vi "Mindsensors LineLeader Config.vi"(10 "Node Data":T1, 11 "NXT":T2) -> ()   [LabVIEW 2010]
uses:
  <vilib>/NXT/Subs/LVHSConnector.ctl
  Datatypes/Node.ctl
  UI Controls/PlugInControls/Pluginbackground.ctl
  <vilib>/Utility/miscctls.llb/LVPointTypeDef.ctl
  ConvertNodeAddrSensor.vi
panel:
  in  "Device Address":u8=2 format="%x"
  out "NXT Port":dbl format="%#.2g"
  out "S 8":dbl
  out "S 7":dbl
  out "S 6":dbl
  out "S 5":dbl
  out "S 4":dbl
  out "S 2":dbl
  out "S 3":dbl
  out "S 1":dbl
  out "XY Graph":cluster{i32[], "data Buffer":u8[]}(graph)
  out "Boolean array":bool[](array[boolean])
  in  "Name":string
  out "Headline":string="Type (auto populated)"
  in  "Sensor parameters":string
  in  "Instance Specific Data":cluster{"Example Data":dbl}
  in  "Reset":bool
  in  "Save":bool
  in  "Stop":bool
  out "Background":T3=TRUE
  # "<- No controls below this line"
  # "Common controls such as Buttons, Rings, Sliders, Graphs, Decorations, etc can be found in the <labview>\\Targets\\NI\\NXT\\NXT Toolkit\\Schematic Editor\\UI Controls\\Plugin Controls\\ folder. Use these controls when possible to ensure a consistent look and feel with LabVIEW Education Edition."
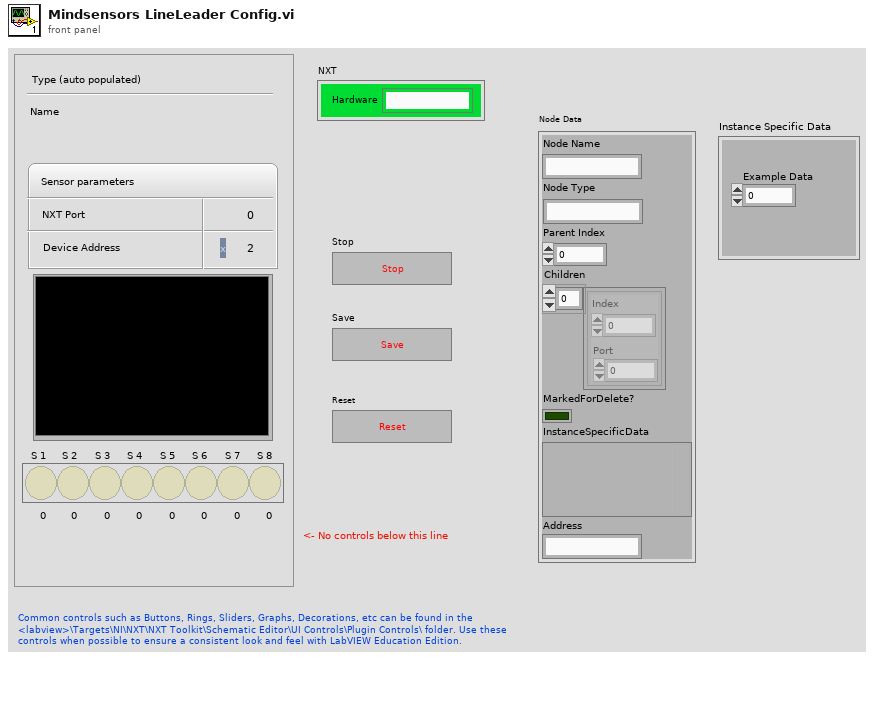
[diagram p1: front panel]
types:
  T1 = typedef "Node.ctl" = cluster{"Node Name":string, "Node Type":string, "Parent Index":i16, "Children":cluster{"Index":u16, "Port":u16}[], "MarkedForDelete?":bool, "InstanceSpecificData":variant, "Address":string}
  T2 = typedef "LVHSConnector.ctl" = cluster{"Hardware":string, "Flattened String":string}
  T3 = typedef "Pluginbackground.ctl" = bool
  T4 = typedef "LVPointTypeDef.ctl" = cluster{"Horizontal":i16, "Vertical":i16}
  T5 = enum8{"Enabled", "Disabled", "Disabled and Grayed Out"}
  T6 = typedef "NXT_InputPort.ctl" = u8
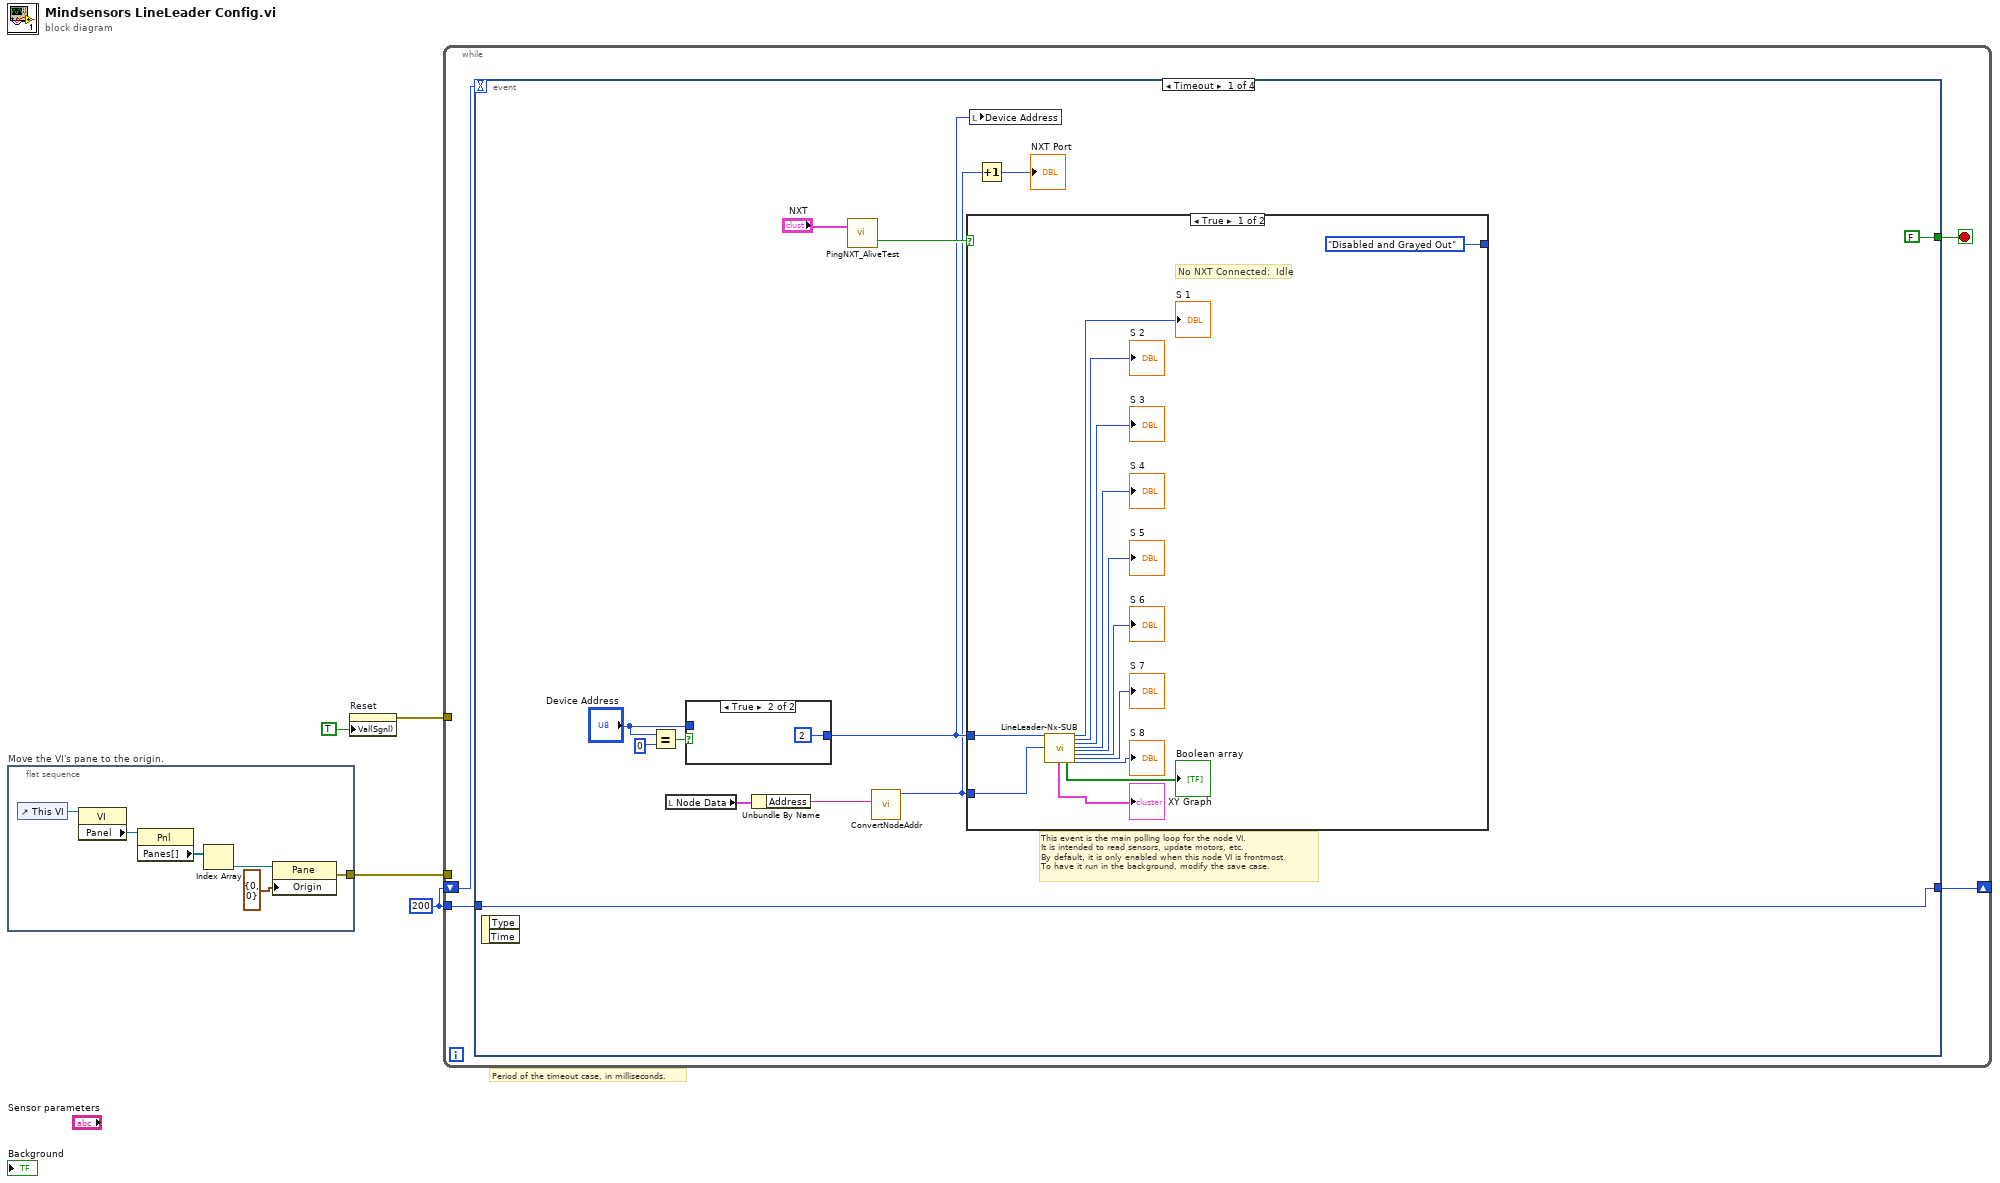
[diagram p0: block diagram]
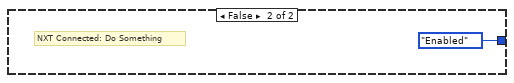
[diagram p3: hidden frame]
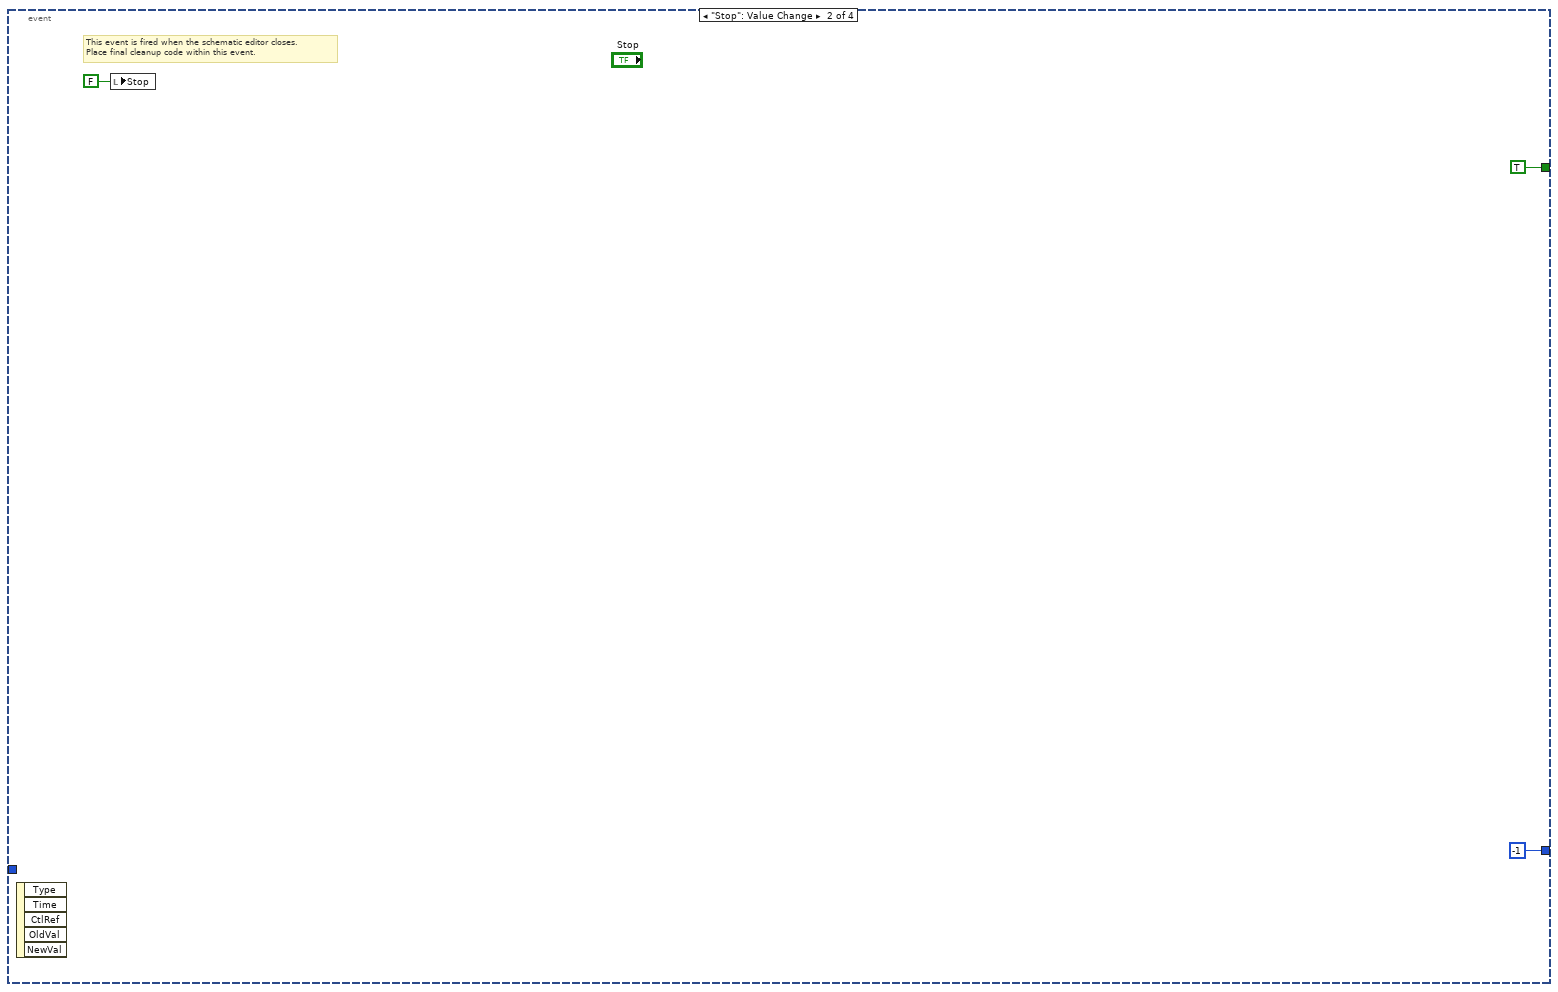
[diagram p4: hidden frame]
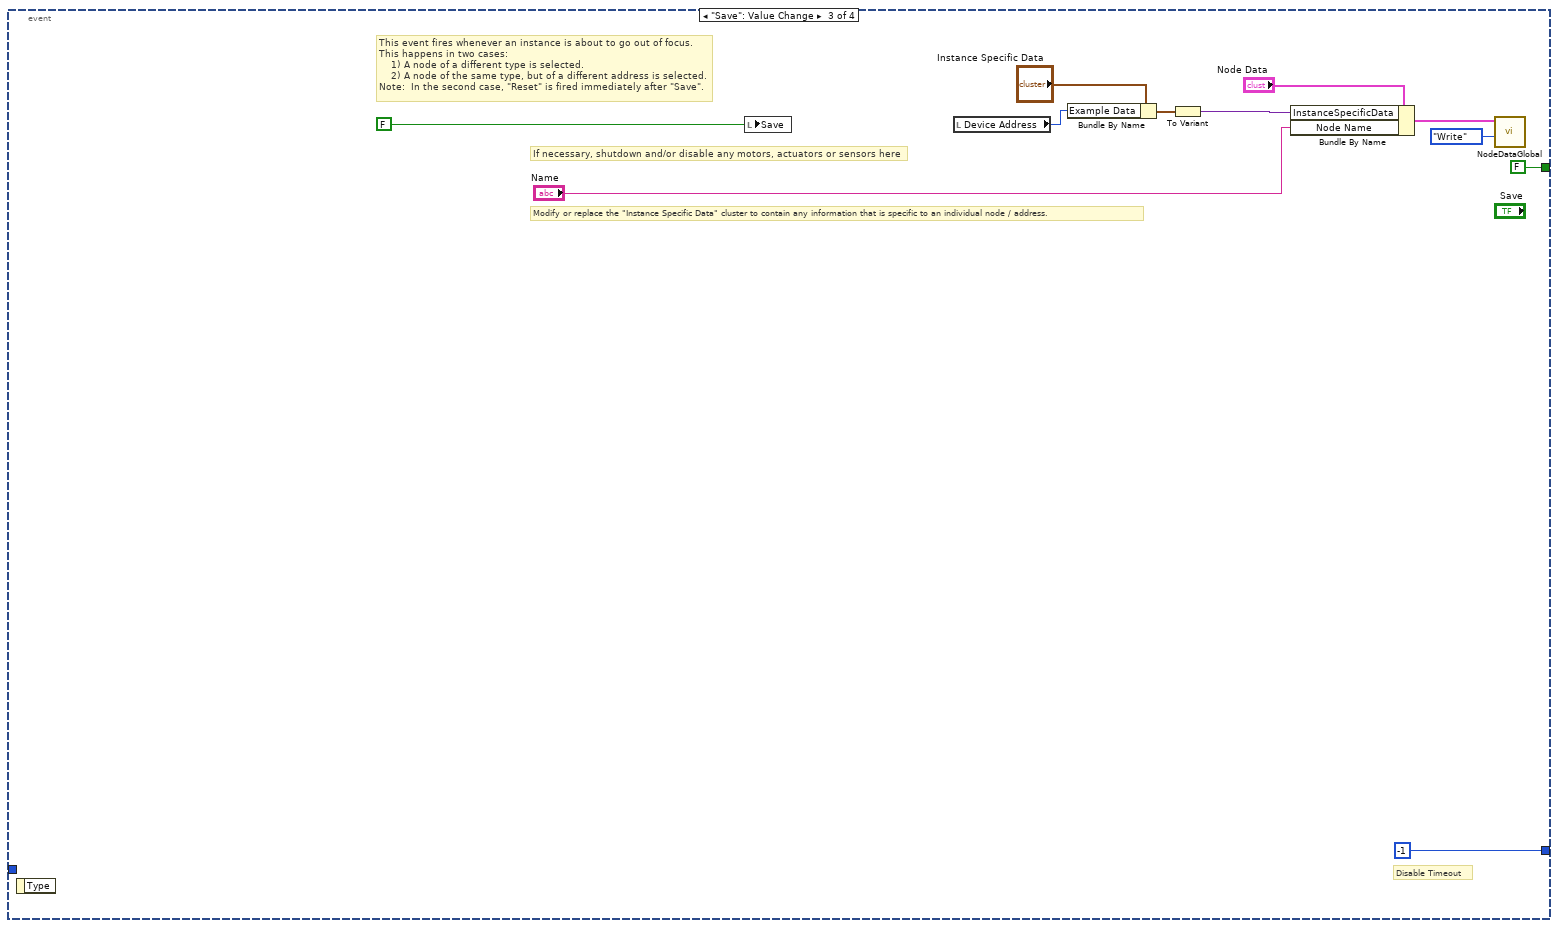
[diagram p5: hidden frame]
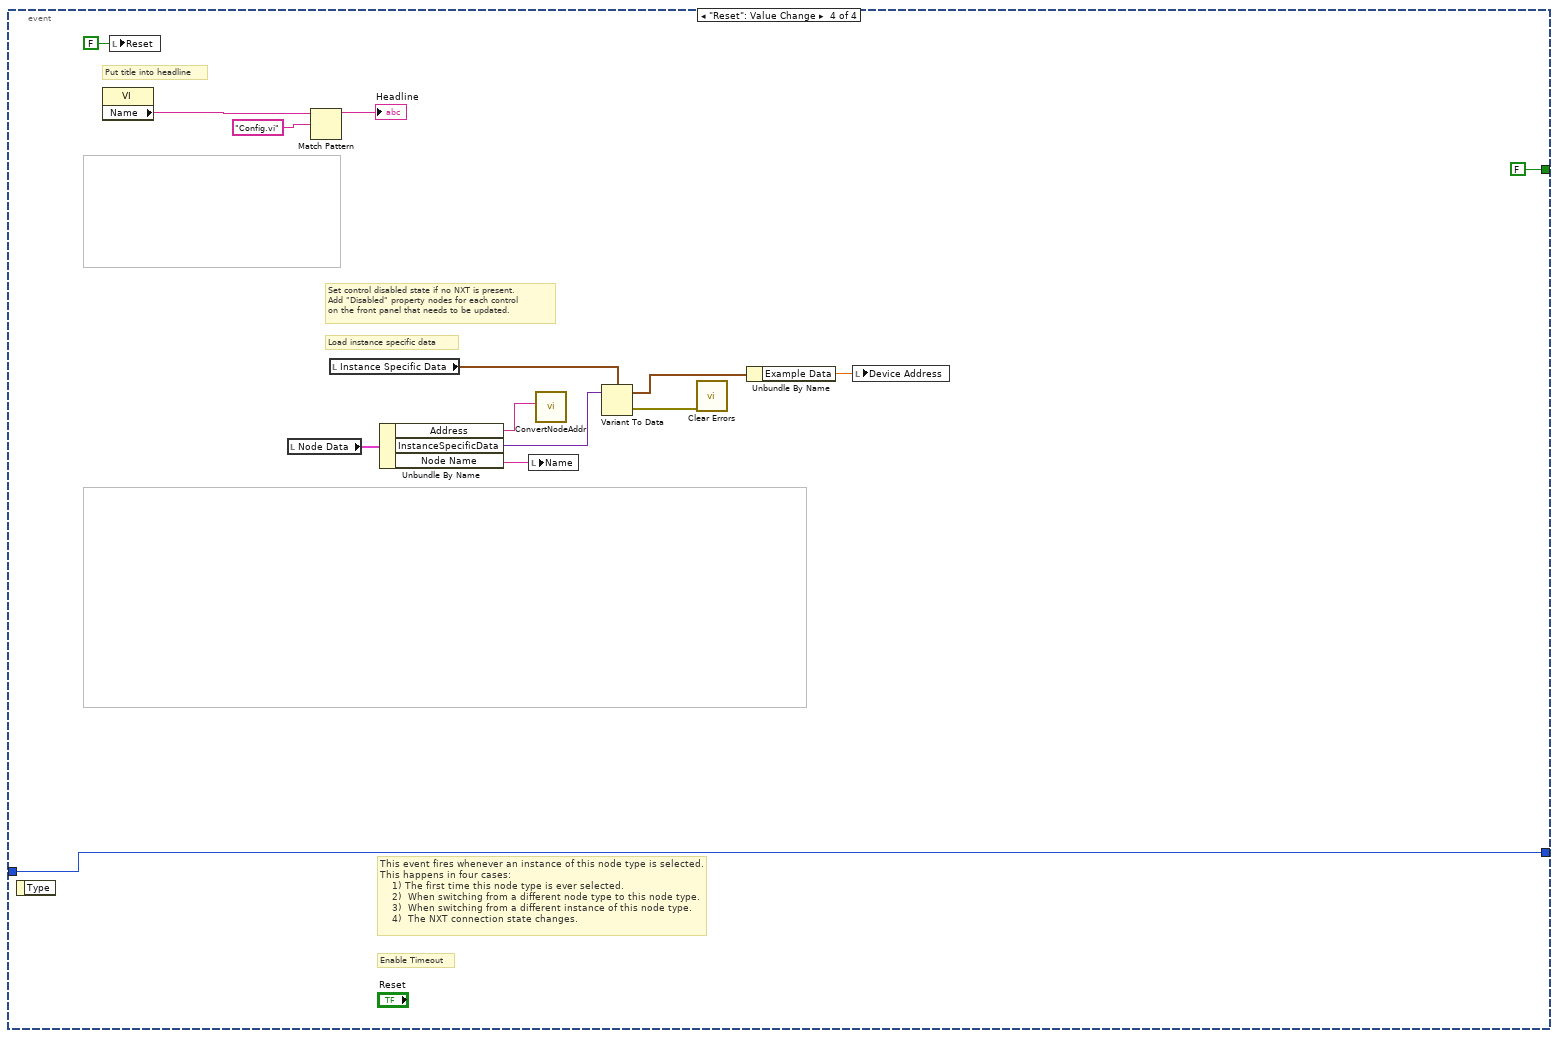
[diagram p6: hidden frame]
diagram:
  w2 = 200
  # "Period of the timeout case, in milliseconds."
  n1 = flat-sequence "Move the VI's pane to the origin." {
    tunnel: [w5] -> w1
    frame #0 {
      n2 = control-ref of="This VI"() -> (w6:refnum<vi>)
      n3 = property class="VI"(reference=w6) -> ("Panel"=w7:refnum<vi>)  [unwired: 1 in, 2 out]
      n4 = property class="Pnl"(reference=w7) -> ("Panes[]"=w8:refnum<vi>[])  [unwired: 1 in, 2 out]
      n5 = Index Array(array=w8) -> (element=w9:refnum<vi>)  [unwired: 1 in]
      n6 = property class="Pane"(reference=w9, "Origin"=T4 {"Horizontal"=0, "Vertical"=0}) -> (error out=w5:errorcluster)  [unwired: 1 in, 1 out]
    }
  }
  n7 = property on="Reset" class="Bool (strict)"("Val(Sgnl)"=TRUE ("Value (Signaling)")) -> (error out=w3:errorcluster)  [unwired: 2 in, 1 out]
  n8 = while {
    tunnel: w3 -> [_]
    shift-right: [w12] -> _
    shift-left: w2 -> [w13]
    tunnel: w2 -> [w11]
    tunnel: w1 -> [_]
    stop <- w14 stop-if-true
    n9 = event shown="[0] Timeout" {
      selector: _ -> [_ _ _ _]
      dyn-events: _ -> [_ _ _ _]
      timeout: w13 -> [_ _ _ _]
      tunnel: [FALSE TRUE FALSE FALSE] -> w14
      tunnel: [w25 -1 -1 w66] -> w12
      tunnel: w11 -> [w25 _ _ w66]
      event Timeout {
        # "This event is the main polling loop for the node VI.\nIt is intended to read sensors, update motors, etc.\nBy default, it is only enabled when this node VI is frontmost.\nTo have it run in the background, modify the save case."
        n10 = event-data() -> ()  [unwired: 1 in, 2 out]
        n11 = Equal?(x="Device Address", y=u8 0) -> (x = y?=w20:bool)
        n12 = local read "Node Data"() -> (w22:T1)
        n13 = case shown="True" w20 {
          tunnel: [w27 u8 2 ("Device Addr 2")] -> w18
          tunnel: "Device Address" -> [w27 _]
          frame False {
          }
          frame True {
          }
        }
        n14 = Unbundle By Name(w22) -> ("Address"=w17:string)
        n15 = call <vilib>:"PingNXT_AliveTest.vi"("NXT"="NXT") -> ("connected?"=w24:bool)  [unwired: 1 in, 1 out]
        n16 = call-poly "ConvertNodeAddr.vi"("Sensor Port"=w17) -> ("NXT Port"=w16:T6)  [unwired: 6 in, 4 out]
        n17 = case shown="True" w24 {
          tunnel: [T5."Disabled and Grayed Out" ("Disabled") T5."Enabled" ("Disabled")] -> _
          tunnel: w16 -> [w30 _]
          tunnel: w18 -> [w29 _]
          frame True {
            # "No NXT Connected:  Idle"
            n18 = call <vilib>:"LineLeader-Nx-SUB.vi"("Select your \nDevice Address"=w29, "Select your \nInput Port"=w30) -> ("XY Graph"=→"XY Graph":cluster{i32[], "data Buffer":u8[]}, "Boolean array"=→"Boolean array":bool[], "S1"=→"S 1":u8, "S2"=→"S 2":u8, "S3"=→"S 3":u8, "S4"=→"S 4":u8, "S5"=→"S 5":u8, "S6"=→"S 6":u8, "S7"=→"S 7":u8, "S8"=→"S 8":u8)  [unwired: 16 in]
          }
          frame False {
            # "NXT Connected: Do Something"
          }
        }
        n19 = local write "Device Address"(w18) -> ()
        n20 = Increment(x=w16) -> (x+1=→"NXT Port":T6)
      }
      event "Stop": Value Change {
        # "This event is fired when the schematic editor closes.\nPlace final cleanup code within this event."
        n21 = event-data() -> ()  [unwired: 1 in, 5 out]
        n22 = local write "Stop"(FALSE ("stop")) -> ()
      }
      event "Save": Value Change {
        # "If necessary, shutdown and/or disable any motors, actuators or sensors here"
        # "Modify or replace the \"Instance Specific Data\" cluster to contain any information that is specific to an individual node / address."
        # "Disable Timeout"
        # "This event fires whenever an instance is about to go out of focus.\nThis happens in two cases:\n    1) A node of a different type is selected.\n    2) A node of the same type, but of a different address is selected.\nNote:  In the second case, \"Reset\" is fired immediately after \"Save\"."
        n23 = event-data() -> ()  [unwired: 1 in, 1 out]
        n24 = local write "Save"(FALSE ("stop")) -> ()
        n25 = local read "Device Address"() -> (w46:u8)
        n26 = Bundle By Name(cluster="Instance Specific Data", "Example Data"=w46) -> (w47:cluster{"Example Data":dbl})
        n27 = To Variant(anything=w47) -> (Variant=w54:variant)
        n28 = Bundle By Name(cluster="Node Data", "InstanceSpecificData"=w54, "Node Name"="Name") -> (w53:T1)
        n29 = call "NodeDataGlobal.vi"("Action"=enum16{"Read", "Write"}."Write", "Node Data In"=w53) -> ()  [unwired: 8 in, 2 out]
      }
      event "Reset": Value Change {
        # "Set control disabled state if no NXT is present.\nAdd \"Disabled\" property nodes for each control\non the front panel that needs to be updated."
        # "Load instance specific data"
        # "Enable Timeout"
        # "This event fires whenever an instance of this node type is selected.\nThis happens in four cases:\n    1) The first time this node type is ever selected.\n    2)  When switching from a different node type to this node type.\n    3)  When switching from a different instance of this node type. \n    4)  The NXT connection state changes."
        # "Put title into headline"
        n30 = event-data() -> ()  [unwired: 1 in, 1 out]
        n31 = property class="VI"() -> ("Name"=w62:string)  [unwired: 2 in, 2 out]
        n32 = local write "Reset"(FALSE ("Reset")) -> ()
        n33 = local read "Node Data"() -> (w67:T1)
        n34 = Match Pattern(string=w62, regular expression="Config.vi") -> (before substring=→"Headline":string)  [unwired: 1 in, 3 out]
        n35 = local read "Instance Specific Data"() -> (w65:cluster{"Example Data":dbl})
        n36 = Unbundle By Name(w67) -> ("Address"=w57:string, "InstanceSpecificData"=w68:variant, "Node Name"=w60:string)
        n37 = local write "Name"(w60) -> ()
        n38 = call-poly "ConvertNodeAddr.vi"("Sensor Port"=w57) -> ()  [unwired: 6 in, 5 out]
        n39 = Variant To Data(Variant=w68, type=w65) -> (error out=w64:errorcluster, data=w59:cluster{"Example Data":dbl})  [unwired: 1 in]
        n40 = call <vilib>:"Clear Errors.vi"("error in (no error)"=w64) -> ()  [unwired: 6 in, 1 out]
        n41 = Unbundle By Name(w59) -> ("Example Data"=w58:dbl)
        n42 = local write "Device Address"(w58) -> ()
      }
    }
  }
